vi "Get Control File Attributes.vi"(8 "error in (no error)":errorcluster, 11 "control file refnum in":refnum<file>) -> (0 "error out":errorcluster, 2 "package attributes":T1={"Package Name"="", "Display name"="", "Version"="", "Display version"="", "Synopsis"="", "Description"="", "Maintainer"="", "Maintainer email address"="", "Category"="", "Homepage"="", "Release notes"="", "Depends"=[], "Recommends"=[], "Suggests"=[], "Conflicts"=[], "Provides"=[], "Replaces"=[], "Supplements"=[], "Enhances"=[], "Product"=FALSE, "User visible"=FALSE, "Installed size (KB)"=0, "Package filesize (bytes)"=0, "Architecture"="", "Agent"="file", "MD5Checksum"=""}, 3 "control file refnum out":refnum<file>)   [LabVIEW 2014, in "NIPM_API.lvlib"]
doc: "Returns the package attributes listed in an unpacked package's control file.\n\nInputs:\nControl file refnum in - This is a file refnum from an unpacked package's control file. Use the Open/Create/Replace File function to open a control file and pass its file refnum to this VI.\n\nOutputs:\nControl file refnum out - Passes the control file refnum out of this VI.\n\nPackage attributes - Returns the package attributes listed in the control file as a cluster."
uses:
  NIPM_API.lvlib
  _support/package attributes.ctl
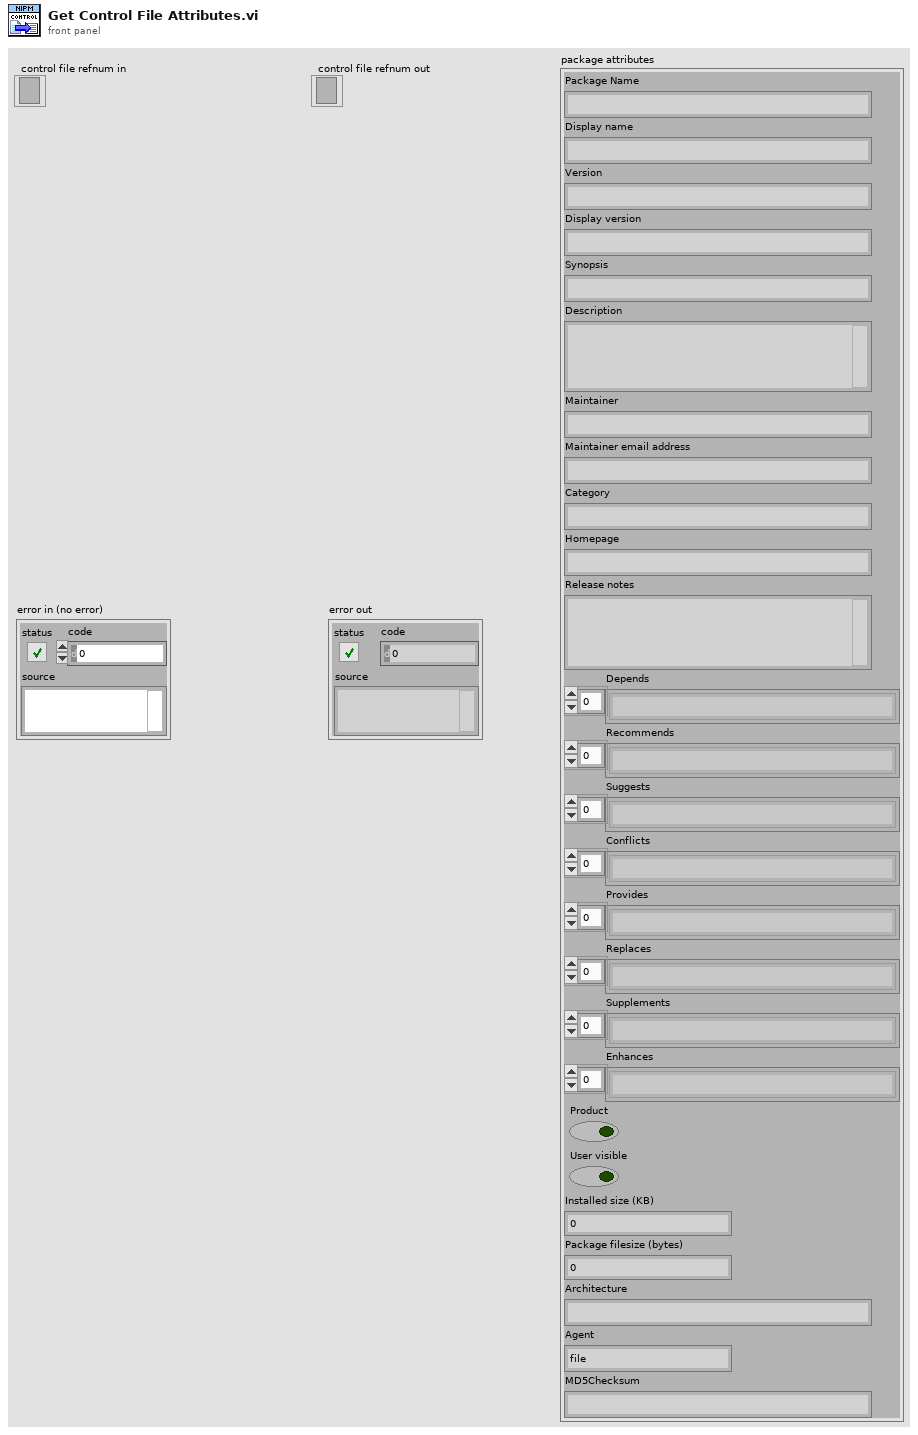
[diagram p1: front panel]
types:
  T1 = typedef "NIPM_API.lvlib/package attributes.ctl" = cluster{"Package Name":string, "Display name":string, "Version":string, "Display version":string, "Synopsis":string, "Description":string, "Maintainer":string, "Maintainer email address":string, "Category":string, "Homepage":string, "Release notes":string, "Depends":string[], "Recommends":string[], "Suggests":string[], "Conflicts":string[], "Provides":string[], "Replaces":string[], "Supplements":string[], "Enhances":string[], "Product":bool, "User visible":bool, "Installed size (KB)":u64, "Package filesize (bytes)":u64, "Architecture":string, "Agent":string, "MD5Checksum":string}
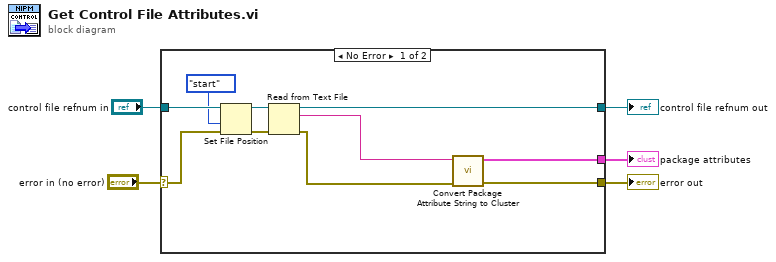
[diagram p0: block diagram]
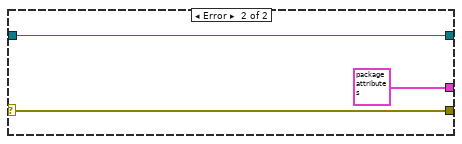
[diagram p2: hidden frame]
diagram:
  n1 = case shown="No Error" "error in (no error)" {
    selector: "error in (no error)" -> [w12 w18]
    tunnel: [w14 T1 {"Package Name"="", "Display name"="", "Version"="", "Display version"="", "Synopsis"="", "Description"="", "Maintainer"="", "Maintainer email address"="", "Category"="", "Homepage"="", "Release notes"="", "Depends"=[], "Recommends"=[], "Suggests"=[], "Conflicts"=[], "Provides"=[], "Replaces"=[], "Supplements"=[], "Enhances"=[], "Product"=FALSE, "User visible"=FALSE, "Installed size (KB)"=0, "Package filesize (bytes)"=0, "Architecture"="", "Agent"="file", "MD5Checksum"=""} ("package attributes")] -> w5
    tunnel: "control file refnum in" -> [w10 w17]
    tunnel: [w13 w17] -> w3
    tunnel: [w6 w18] -> w1
    frame No Error {
      n2 = Set File Position(refnum=w10, from (0:start)=enum16{"start", "end", "current"}."start", error in=w12) -> (refnum out=w9:refnum<file>, error out=w11:errorcluster)  [unwired: 1 in]
      n3 = Read from Text File(file (use dialog)=w9, error in=w11) -> (refnum out=w13:refnum<file>, text=w15:string, error out=w7:errorcluster)  [unwired: 2 in, 1 out]
      n4 = call "Convert Package Attribute String to Cluster.vi"("error in (no error)"=w7, "nipkg CLI info string"=w15) -> ("error out"=w6:errorcluster, "package attributes"=w14:T1)  [unwired: 8 in]
    }
    frame Error {
    }
  }
  "package attributes" <- w5
  "control file refnum out" <- w3
  "error out" <- w1
